vi "processing calibration.vi"() -> ()   [LabVIEW 2019, in "Calibration Lib.lvlib"]
uses:
  Calibration Lib.lvlib
  <vilib>/vision/Image Controls.llb/IMAQ Image.ctl
  <vilib>/Utility/miscctls.llb/LVRowAndColumnTypeDef.ctl
  <vilib>/Analysis/Matrix/Numeric/Conversions/Array To Matrix - RA2.vi
  <vilib>/addons/Multicore Analysis and Sparse Matrix/Linear Algebra/_linalg/Solve Least Squares Problems (DBL).vi
  <vilib>/addons/database/Connection.llb/DB Tools Open Connec (String).vi
  database.lvlib
  <vilib>/addons/database/NI_Database_API.lvlib
  <vilib>/addons/Multicore Analysis and Sparse Matrix/Linear Algebra/NI_MASM_BasicLinAlg.lvlib
  <vilib>/Analysis/Matrix/NI_Matrix.lvlib
panel:
  out "calibration factors":dbl[](array[numeric])
  out "calibration Matrix":dbl[][](array[numeric])
  in  "Tab Control":enum32{"img 1", "img2", "img3"}(tab)
  out "Image":T1(plugin-control)
  out "Image 3":T1(plugin-control)
  out "Image 4":T1(plugin-control)
  out "Error out 2":errorcluster
  in  "Delete":bool
  out "error out":errorcluster
  out "data":string[][](array[string])
  out "Calibration String":string
  in  "Close":bool
  in  "Calibrate":bool caption="Saving txt"
  out "Processing Table":string[][](table)
  in  "Disc Number":string(combo)
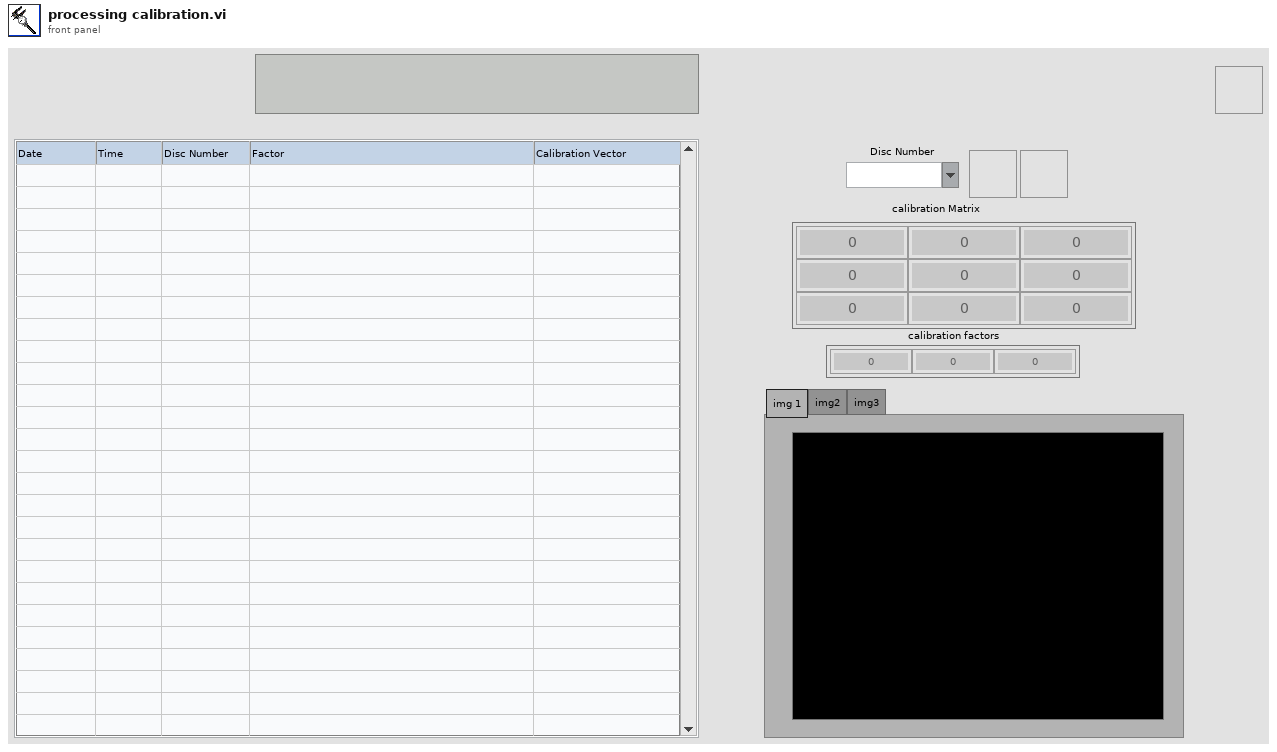
[diagram p1: front panel]
types:
  T1 = typedef "IMAQ Image.ctl" = refnum<image>
  T2 = typedef "LVRowAndColumnTypeDef.ctl" = cluster{"Row":i32, "Column":i32}
  T3 = typedef "NI_Matrix.lvlib/RealMatrix.ctl" = dbl[][]
  T4 = cluster{"date/time string":string, "date/time string":string, i32, "spreadsheet string":string}
  T5 = cluster{i32, "date/time string":string, "date/time string":string, string}
  T6 = typedef "NI_Database_API.lvlib/Conn ObjectReference.ctl" = refnum<k1>
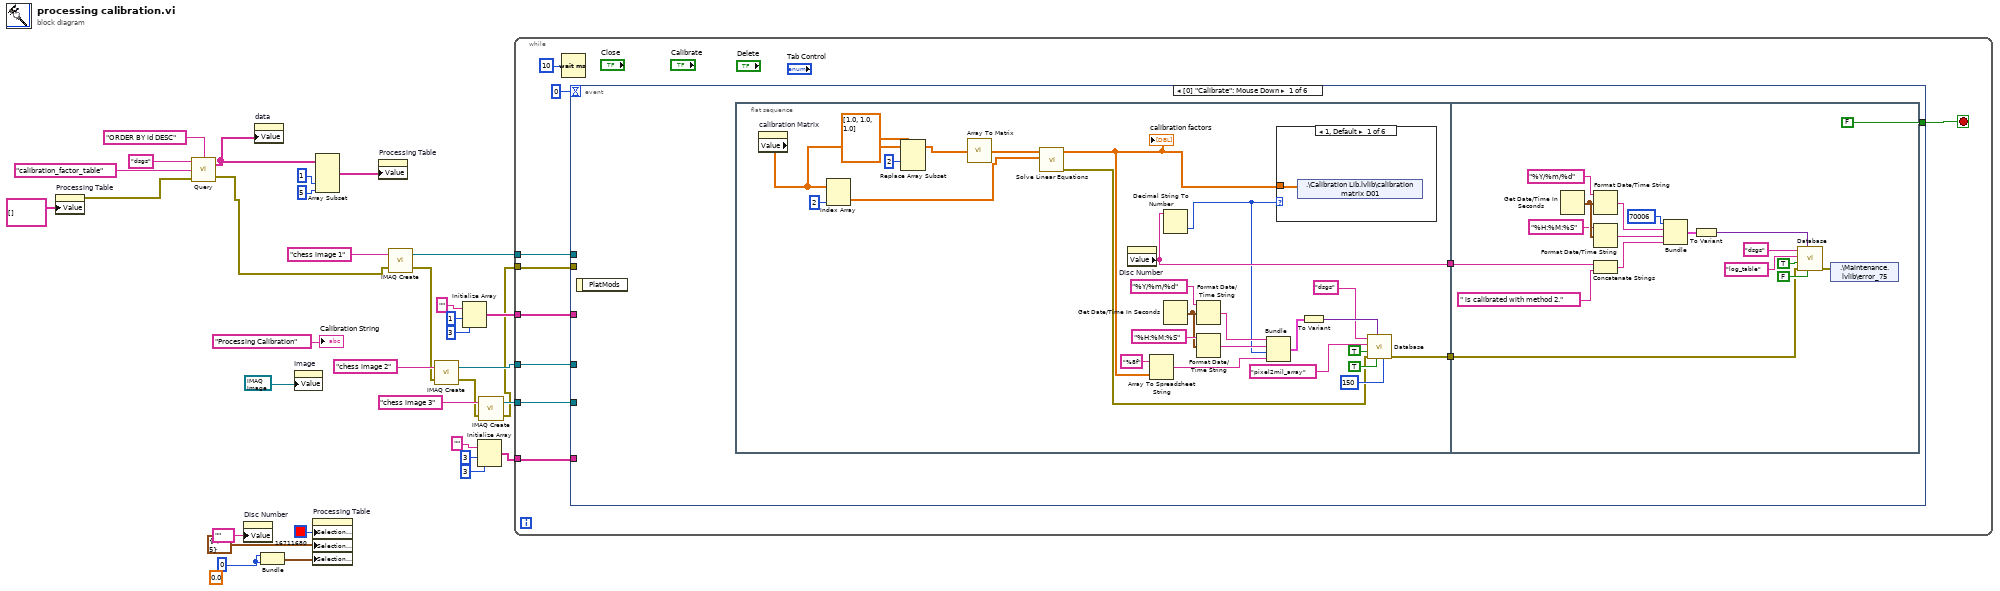
[diagram p0: block diagram]
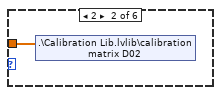
[diagram p2: hidden frame]
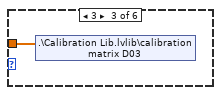
[diagram p3: hidden frame]
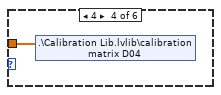
[diagram p4: hidden frame]
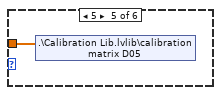
[diagram p5: hidden frame]
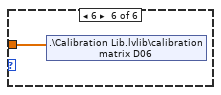
[diagram p6: hidden frame]
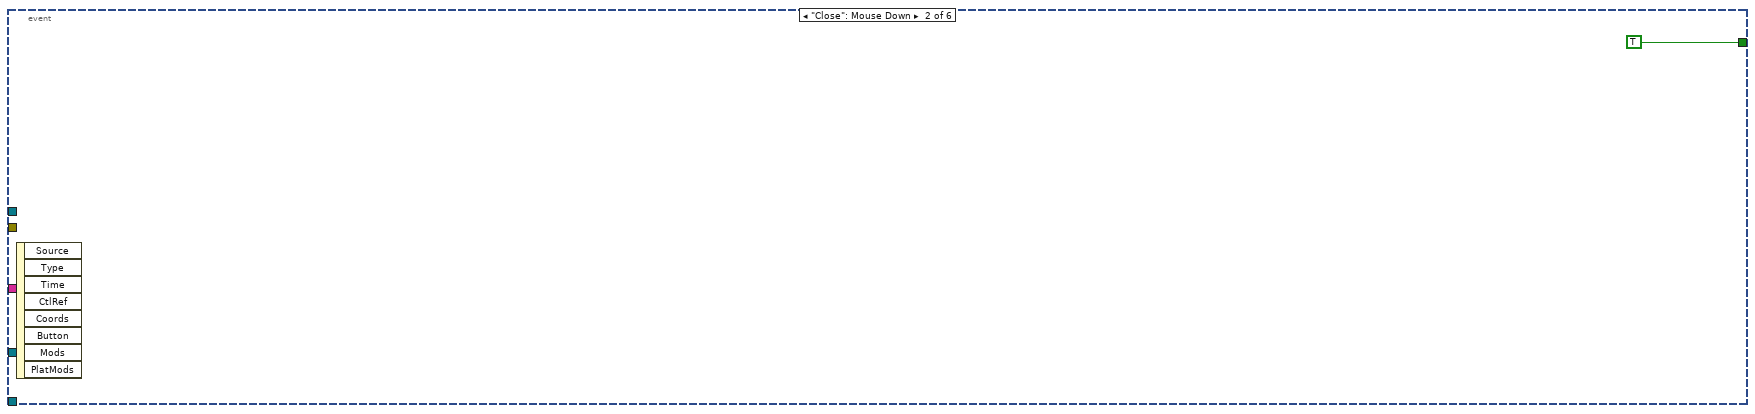
[diagram p7: hidden frame]
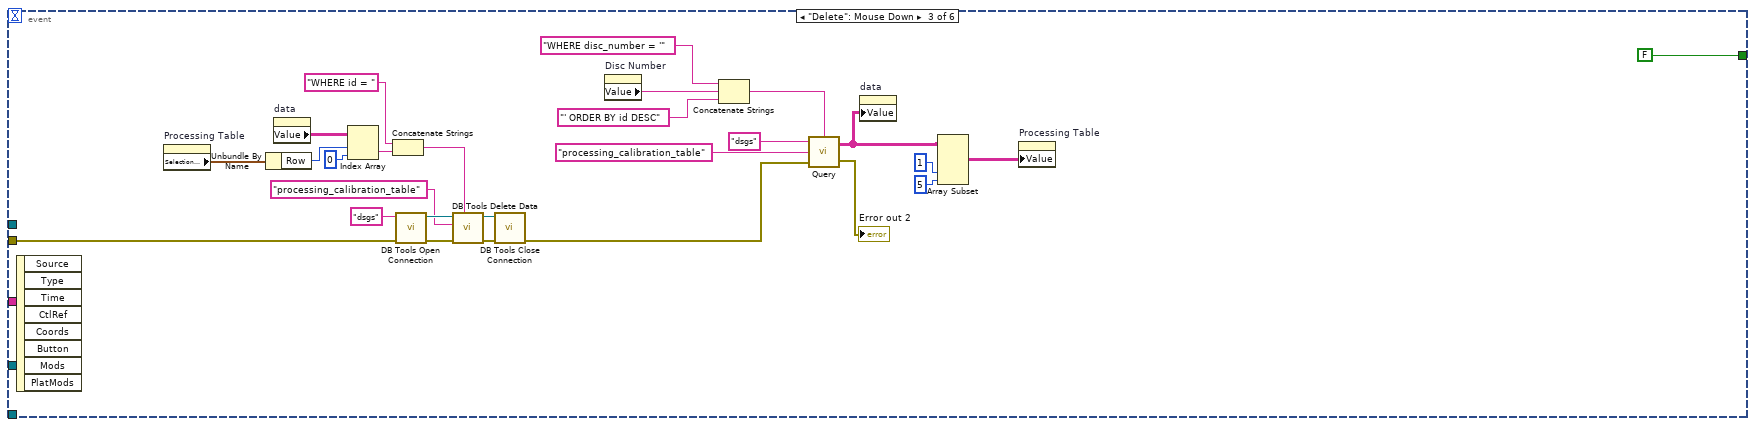
[diagram p8: hidden frame]
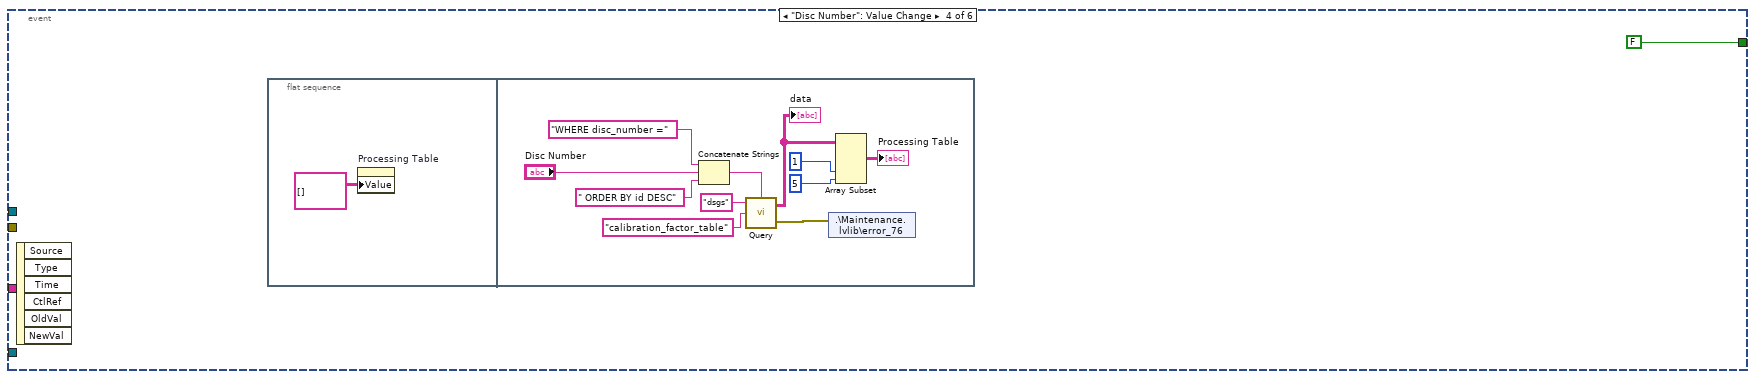
[diagram p9: hidden frame]
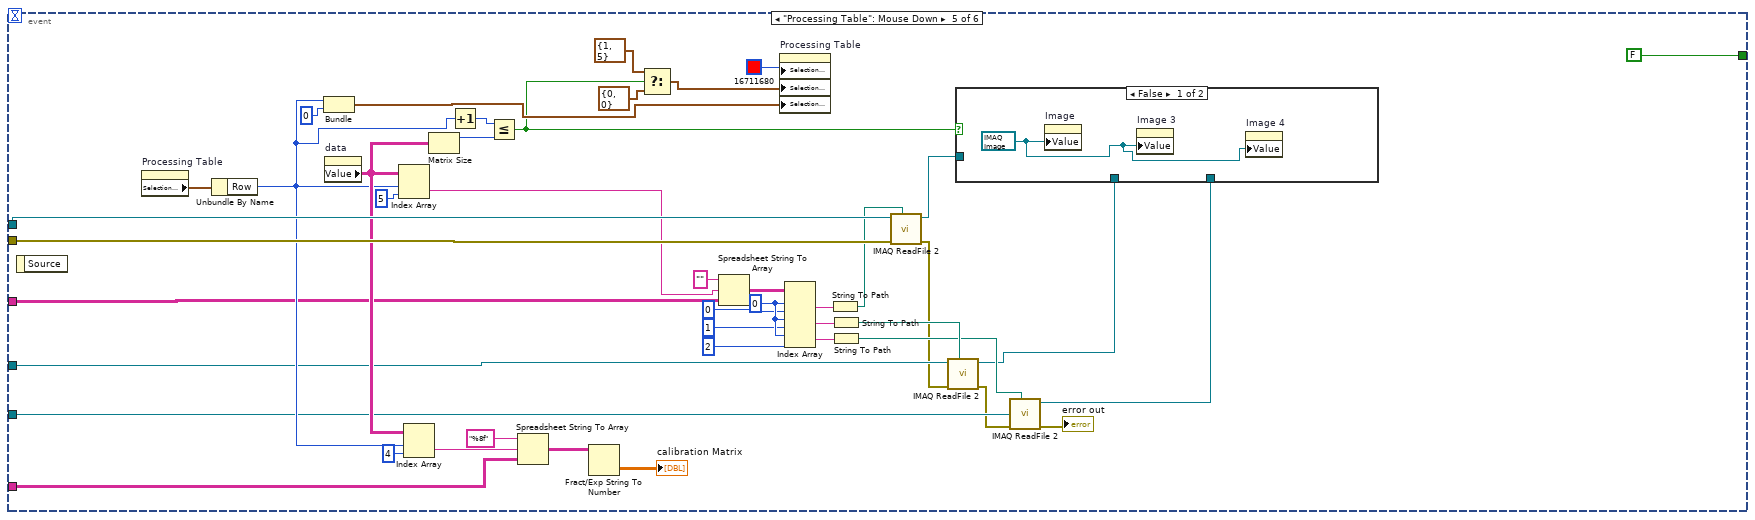
[diagram p10: hidden frame]
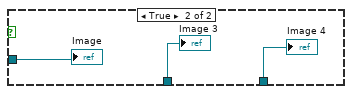
[diagram p11: hidden frame]
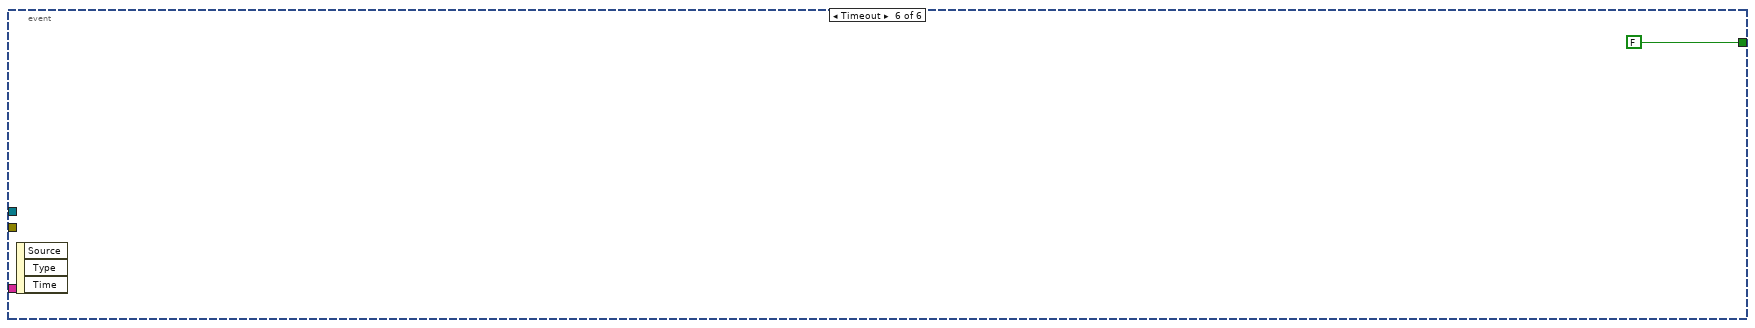
[diagram p12: hidden frame]
diagram:
  w18 = 0 ("Row")
  (unwired) sgl 0.0 ("Calibration Factor")
  n1 = property on="Processing Table" class="Tbl (strict)"("Value"=string[][] []) -> (error out=w17:errorcluster)  [unwired: 2 in, 1 out]
  n2 = call "Query.vi"("Condition"="ORDER BY id DESC", "Error in"=w17, "Table Name"="calibration_factor_table", "Connection Name"="dsgs") -> ("Error out"=w1:errorcluster, "data"=w24:string[][])
  n3 = property on="Disc Number" class="CmbBox"("Value"="" ("Disc Number")) -> ()  [unwired: 2 in, 2 out]
  n4 = property on="data" class="Arr (strict)"("Value"=w24) -> ()  [unwired: 2 in, 2 out]
  n5 = Bundle("Row"=w18, "Row"=w18) -> (w19:cluster{"Row":i32, "Row":i32})  [unwired: 1 in]
  n6 = property on="Image" class="ImageControl"("Value"=T1 refnum ("Image Out")) -> ()  [unwired: 2 in, 2 out]
  n7 = property on="Processing Table" class="Tbl (strict)"("Selection Color"=u32 16711680, "Selection Size"=T2 {"Row"=1, "Column"=5}, "Selection Start"=w19) -> ()  [unwired: 2 in, 2 out]
  n8 = Array Subset(array=w24, index (col)=1 ("index"), length (col)=5 ("length")) -> (w25:string[][])  [unwired: 2 in]
  n9 = property on="Processing Table" class="Tbl (strict)"("Value"=w25) -> ()  [unwired: 2 in, 2 out]
  n10 = call "IMAQ Create"("Image Name"="chess image 1", "error in (no error)"=w1) -> ("New Image"=w32:T1, "error out"=w9:errorcluster)  [unwired: 3 in]
  n11 = call "IMAQ Create"("Image Name"="chess image 2", "error in (no error)"=w9) -> ("New Image"=w11:T1, "error out"=w8:errorcluster)  [unwired: 3 in]
  n12 = Initialize Array("", 1 ("dimension size"), 3 ("dimension size")) -> (w14:string[][])
  n13 = Initialize Array("", 3 ("dimension size"), 3 ("dimension size")) -> (w2:string[][])
  n14 = call "IMAQ Create"("Image Name"="chess image 3", "error in (no error)"=w8) -> ("New Image"=w10:T1, "error out"=w7:errorcluster)  [unwired: 3 in]
  n15 = while {
    tunnel: w32 -> [w40]
    tunnel: w7 -> [w39]
    tunnel: w14 -> [w38]
    tunnel: w11 -> [w37]
    tunnel: w10 -> [w36]
    tunnel: w2 -> [w35]
    stop <- w42 stop-if-true
    n16 = Wait (ms)(milliseconds to wait=u32 10) -> ()  [unwired: 1 out]
    n17 = event shown="[0] \"Calibrate\": Mouse Down" {
      selector: _ -> [_ _ _ _ _ _]
      dyn-events: _ -> [_ _ _ _ _ _]
      timeout: 0 -> [_ _ _ _ _ _]
      tunnel: [FALSE TRUE FALSE FALSE FALSE FALSE] -> w42
      tunnel: w40 -> [_ _ _ _ w179 _]
      tunnel: w39 -> [_ _ w110 _ w178 _]
      tunnel: w38 -> [_ _ _ _ w140 _]
      tunnel: w37 -> [_ _ _ _ w150 _]
      tunnel: w36 -> [_ _ _ _ w149 _]
      tunnel: w35 -> [_ _ _ _ w139 _]
      event "Calibrate": Mouse Down {
        n18 = event-data() -> ()  [unwired: 1 in, 1 out]
        n19 = flat-sequence {
          tunnel: [w65] -> w45
          tunnel: [w48] -> w44
          tunnel: w45 -> [w83]
          tunnel: w44 -> [w79]
          frame #0 {
            n20 = property on="calibration Matrix" class="Arr (strict)"() -> ("Value"=w70:dbl[][])  [unwired: 2 in, 2 out]
            n21 = Index Array(array=w70, index (col)=2 ("disabled index (col)")) -> (element=w66:dbl[])  [unwired: 1 in]
            n22 = Replace Array Subset(array=w70, new element=dbl[] [1.0, 1.0, 1.0] ("new element/subarray"), index (col)=2 ("disabled index (col)")) -> (w68:dbl[][])  [unwired: 1 in]
            n23 = call-poly <vilib>:"Array To Matrix.vi"("Real 2D Array"=w68) -> ("Real Matrix"=w67:T3)
            n24 = call-poly <vilib>:"Solve Linear Equations.vi"("Known Vector"=w66, "Input Matrix"=w67) -> ("error out"=w47:errorcluster, "Solution Vector"=w58:dbl[])  [unwired: 8 in]
            "calibration factors" <- w58
            n25 = property on="Disc Number" class="CmbBox"() -> ("Value"=w65:string)  [unwired: 2 in, 2 out]
            n26 = Array To Spreadsheet String(array=w58, 3:"%8f" ("format string")) -> (spreadsheet string=w57:string)  [unwired: 1 in]
            n27 = Get Date/Time In Seconds() -> (seconds since 1Jan1904=w62:timestamp)
            n28 = Decimal String To Number(string=w65) -> (number=w59:i32)  [unwired: 2 in, 1 out]
            n29 = Format Date/Time String(time format string (%c)="%Y/%m/%d", seconds (now)=w62) -> (date/time string=w61:string)  [unwired: 1 in]
            n30 = Format Date/Time String(time format string (%c)="%H:%M:%S", seconds (now)=w62) -> (date/time string=w60:string)  [unwired: 1 in]
            n31 = Bundle("date/time string"=w61, "date/time string"=w60, w59, "spreadsheet string"=w57) -> (w56:T4)  [unwired: 1 in]
            n32 = case shown="1, Default" w59 {
              tunnel: w58 -> [w73 w74 w75 w76 w77 w78]
              frame 1, Default {
                n33 = shared-variable ".\\Calibration Lib.lvlib\\calibration matrix D01"(w73) -> ()  [unwired: 1 in, 1 out]
              }
              frame 2 {
                n34 = shared-variable ".\\Calibration Lib.lvlib\\calibration matrix D02"(w74) -> ()  [unwired: 1 in, 1 out]
              }
              frame 3 {
                n35 = shared-variable ".\\Calibration Lib.lvlib\\calibration matrix D03"(w75) -> ()  [unwired: 1 in, 1 out]
              }
              frame 4 {
                n36 = shared-variable ".\\Calibration Lib.lvlib\\calibration matrix D04"(w76) -> ()  [unwired: 1 in, 1 out]
              }
              frame 5 {
                n37 = shared-variable ".\\Calibration Lib.lvlib\\calibration matrix D05"(w77) -> ()  [unwired: 1 in, 1 out]
              }
              frame 6 {
                n38 = shared-variable ".\\Calibration Lib.lvlib\\calibration matrix D06"(w78) -> ()  [unwired: 1 in, 1 out]
              }
            }
            n39 = To Variant(anything=w56) -> (Variant=w55:variant)
            n40 = call "Database.vi"("Maximum Row"=150, "Delete row?"=TRUE, "Data"=w55, "Error in"=w47, "Auto Increment ID?"=TRUE, "Table"="pixel2mil_array", "Connection"="dsgs") -> ("Error out"=w48:errorcluster)  [unwired: 4 in]
          }
          frame #1 {
            n41 = Get Date/Time In Seconds() -> (seconds since 1Jan1904=w91:timestamp)
            n42 = Format Date/Time String(time format string (%c)="%Y/%m/%d", seconds (now)=w91) -> (date/time string=w92:string)  [unwired: 1 in]
            n43 = Format Date/Time String(time format string (%c)="%H:%M:%S", seconds (now)=w91) -> (date/time string=w93:string)  [unwired: 1 in]
            n44 = Concatenate Strings(w83, " is calibrated with method 2." ("string")) -> (w81:string)
            n45 = Bundle(70006, "date/time string"=w92, "date/time string"=w93, w81) -> (w94:T5)  [unwired: 1 in]
            n46 = To Variant(anything=w94) -> (Variant=w95:variant)
            n47 = call "Database.vi"("Delete row?"=FALSE, "Data"=w95, "Error in"=w79, "Auto Increment ID?"=TRUE, "Table"="log_table" ("table"), "Connection"="dsgs" ("table")) -> ("Error out"=w80:errorcluster)  [unwired: 5 in]
            n48 = shared-variable ".\\Maintenance.lvlib\\error_75"(w80) -> ()  [unwired: 1 in, 1 out]
          }
        }
      }
      event "Close": Mouse Down {
        n49 = event-data() -> ()  [unwired: 1 in, 8 out]
      }
      event "Delete": Mouse Down {
        n50 = event-data() -> ()  [unwired: 1 in, 8 out]
        n51 = property on="Processing Table" class="Tbl (strict)"() -> ("Selection Start"=w121:T2)  [unwired: 2 in, 2 out]
        n52 = Unbundle By Name(w121) -> ("Row"=w123:i32)
        n53 = property on="data" class="Arr (strict)"() -> ("Value"=w122:string[][])  [unwired: 2 in, 2 out]
        n54 = Index Array(array=w122, index (row)=w123, index (col)=0 ("disabled index (col)")) -> (element=w115:string)
        n55 = Concatenate Strings("WHERE id = " ("string"), w115) -> (w113:string)
        n56 = call-poly <vilib>:"DB Tools Open Connection.vi"("error in (no error)"=w110, "connection information"="dsgs") -> ("error out"=w116:errorcluster, "connection reference"=w118:T6)  [unwired: 6 in]
        n57 = call <vilib>:"DB Tools Delete Data.vi"("condition"=w113, "error in (no error)"=w116, "table"="processing_calibration_table", "connection reference"=w118) -> ("error out"=w112:errorcluster, "connection reference out"=w111:T6)  [unwired: 6 in]
        n58 = call <vilib>:"DB Tools Close Connection.vi"("error in (no error)"=w112, "connection reference"=w111) -> ("error out"=w107:errorcluster)  [unwired: 5 in]
        n59 = property on="Disc Number" class="CmbBox"() -> ("Value"=w97:string)  [unwired: 2 in, 2 out]
        n60 = Concatenate Strings("WHERE disc_number = '" ("string"), w97, "' ORDER BY id DESC" ("Condition")) -> (w99:string)
        n61 = call "Query.vi"("Condition"=w99, "Error in"=w107, "Table Name"="processing_calibration_table", "Connection Name"="dsgs") -> ("Error out"=→"Error out 2":errorcluster, "data"=w103:string[][])
        n62 = property on="data" class="Arr (strict)"("Value"=w103) -> ()  [unwired: 2 in, 2 out]
        n63 = Array Subset(array=w103, index (col)=1 ("index"), length (col)=5 ("length")) -> (w106:string[][])  [unwired: 2 in]
        n64 = property on="Processing Table" class="Tbl (strict)"("Value"=w106) -> ()  [unwired: 2 in, 2 out]
      }
      event "Disc Number": Value Change {
        n65 = event-data() -> ()  [unwired: 1 in, 6 out]
        n66 = flat-sequence {
          frame #0 {
            n67 = property on="Processing Table" class="Tbl (strict)"("Value"=string[][] []) -> ()  [unwired: 2 in, 2 out]
          }
          frame #1 {
            n68 = Concatenate Strings("WHERE disc_number =", "Disc Number", " ORDER BY id DESC" ("string")) -> (w135:string)
            n69 = call "Query.vi"("Condition"=w135, "Table Name"="calibration_factor_table", "Connection Name"="dsgs") -> ("Error out"=w126:errorcluster, "data"=w136:string[][])  [unwired: 1 in]
            "data" <- w136
            n70 = shared-variable ".\\Maintenance.lvlib\\error_76"(w126) -> ()  [unwired: 1 in, 1 out]
            n71 = Array Subset(array=w136, index (col)=1 ("index"), length (col)=5 ("length")) -> (→"Processing Table":string[][])  [unwired: 2 in]
          }
        }
      }
      event "Processing Table": Mouse Down {
        w160 = 0 ("index (row)")
        n72 = event-data() -> ()  [unwired: 1 in, 1 out]
        n73 = property on="Processing Table" class="Tbl (strict)"() -> ("Selection Start"=w180:T2)  [unwired: 2 in, 2 out]
        n74 = Unbundle By Name(w180) -> ("Row"=w169:i32)
        n75 = Bundle("Row"=w169, "Row"=0) -> (w174:cluster{"Row":i32, "Row":i32})  [unwired: 1 in]
        n76 = property on="data" class="Arr (strict)"() -> ("Value"=w172:string[][])  [unwired: 2 in, 2 out]
        n77 = Index Array(array=w172, index (row)=w169, index (col)=5 ("disabled index (col)")) -> (element=w162:string)
        n78 = Index Array(array=w172, index (row)=w169, index (col)=4 ("disabled index (col)")) -> (element=w141:string)
        n79 = Matrix Size(0:w172) -> (1:w171:i32)  [unwired: 1 out]
        n80 = Increment(x=w169) -> (x+1=w170:i32)
        n81 = Less Or Equal?(x=w170, y=w171) -> (x <= y?=w167:bool)
        n82 = Spreadsheet String To Array(format string="%8f", spreadsheet string=w141, array type (2D Dbl)=w139) -> (array=w138:string[][])  [unwired: 1 in]
        n83 = Fract/Exp String To Number(string=w138) -> (number=→"calibration Matrix":dbl[][])  [unwired: 3 in, 1 out]
        n84 = Select(t=T2 {"Row"=1, "Column"=5} ("Selection Size"), s=w167, f=T2 {"Row"=0, "Column"=0}) -> (s? t:f=w165:T2)
        n85 = Spreadsheet String To Array(format string="", spreadsheet string=w162, array type (2D Dbl)=w140) -> (array=w161:string[][])  [unwired: 1 in]
        n86 = property on="Processing Table" class="Tbl (strict)"("Selection Color"=u32 16711680, "Selection Size"=w165, "Selection Start"=w174) -> ()  [unwired: 2 in, 2 out]
        n87 = Index Array(array=w161, index (row) #1=w160, index (col) #1=0 ("disabled index (col)"), index (row) #2=w160, index (col) #2=1 ("disabled index (col)"), index (row) #3=w160, index (col) #3=2 ("disabled index (col)")) -> (element #1=w156:string, element #2=w155:string, element #3=w154:string)
        n88 = String To Path(string=w156) -> (path=w153:path)
        n89 = String To Path(string=w155) -> (path=w152:path)
        n90 = String To Path(string=w154) -> (path=w151:path)
        n91 = call "IMAQ ReadFile 2"("File Path"=w153, "error in (no error)"=w178, "Image"=w179) -> ("error out"=w148:errorcluster, "Image Out"=w168:T1)  [unwired: 4 in, 3 out]
        n92 = call "IMAQ ReadFile 2"("File Path"=w152, "error in (no error)"=w148, "Image"=w150) -> ("error out"=w147:errorcluster, "Image Out"=w145:T1)  [unwired: 4 in, 3 out]
        n93 = call "IMAQ ReadFile 2"("File Path"=w151, "error in (no error)"=w147, "Image"=w149) -> ("error out"=→"error out":errorcluster, "Image Out"=w144:T1)  [unwired: 4 in, 3 out]
        n94 = case shown="False" w167 {
          tunnel: w168 -> [_ w184]
          tunnel: w145 -> [_ w183]
          tunnel: w144 -> [_ w182]
          frame False {
            w181 = T1 refnum ("Image Out")
            n95 = property on="Image" class="ImageControl"("Value"=w181) -> ()  [unwired: 2 in, 2 out]
            n96 = property on="Image 3" class="ImageControl"("Value"=w181) -> ()  [unwired: 2 in, 2 out]
            n97 = property on="Image 4" class="ImageControl"("Value"=w181) -> ()  [unwired: 2 in, 2 out]
          }
          frame True {
            "Image" <- w184
            "Image 3" <- w183
            "Image 4" <- w182
          }
        }
      }
      event Timeout {
        n98 = event-data() -> ()  [unwired: 1 in, 3 out]
      }
    }
  }
  "Calibration String" <- "Processing Calibration" ("Calibration String")
